vi "RWA_PC File Write String.vi"(8 "Error":errorcluster, 9 "String":string, 11 "Path":path) -> (0 "Error Out":errorcluster, 3 "Path Out":path)   [LabVIEW 2023]
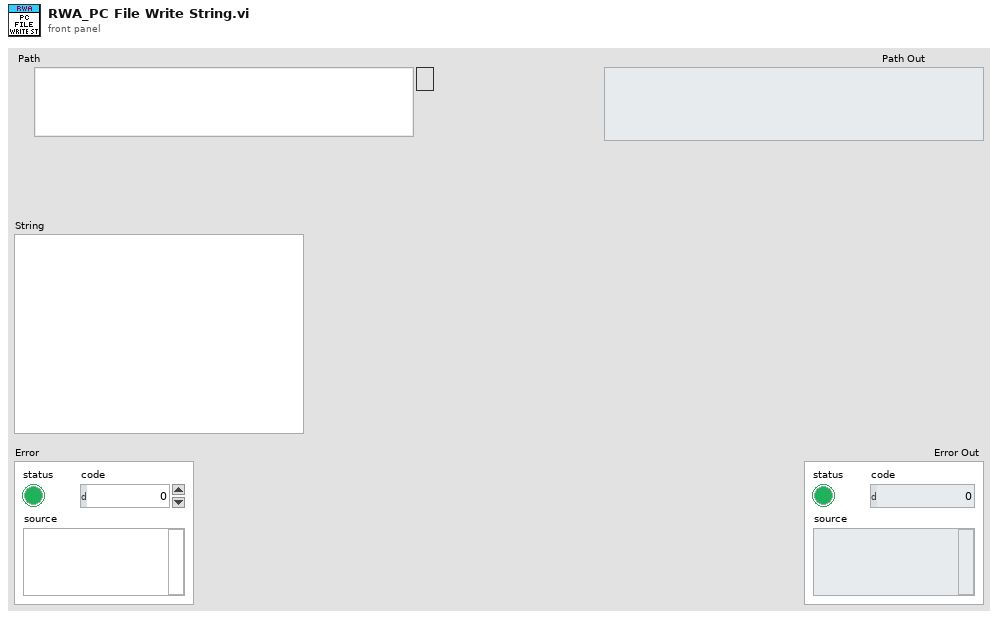
[diagram p1: front panel]
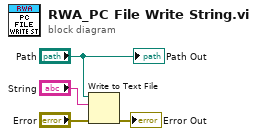
[diagram p0: block diagram]
diagram:
  n1 = Write to Text File(file (use dialog)="Path", text="String", error in="Error") -> (error out=→"Error Out":errorcluster)  [unwired: 3 out]
  "Path Out" <- "Path"
